vi "Timer1 Callback.vi"   [LabVIEW 2014]
doc: "Callback VI for the timer interrupt."
uses:
  <vilib>/Aledyne-TSXperts/Arduino Compatible Compiler for LabVIEW/Arduino Compatible Compiler for LabVIEW.lvlib
  Timer1/Timer1.lvlib
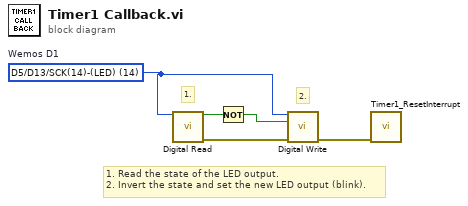
[diagram p0: block diagram]
diagram:
  w1 = u8 14 items=["D0-RX(3)"=3, "D1-TX(1)"=1, "D2(16)"=16, "D3/D15/SCL(5)"=5, "D4/D14/SDA(4)"=4, "D5/D13/SCK(14)-(LED)"=14, "D6/D12/MISO(12)"=12, "D7/D11/MOSI(13)"=13, "D8(0)"=0, "D9/TX1(2)"=2, "D10/SS (15)"=15, "ADC0,(17)"=17]  # Wemos D1
  # "2."
  # "1."
  # "1. Read the state of the LED output.\n2. Invert the state and set the new LED output (blink)."
  n1 = call <vilib>:"Digital Read.vi"("pin"=w1) -> ("state"=w5:bool, "error out"=w3:errorcluster)  [unwired: 13 in]
  n2 = Not(x=w5) -> (.not. x?=w4:bool)
  n3 = call <vilib>:"Digital Write.vi"("pin"=w1, "state"=w4, "error in (no error)"=w3) -> ("error out"=w2:errorcluster)  [unwired: 12 in]
  n4 = call "Timer1_ResetInterrupt.vi"("error in"=w2) -> ()  [unwired: 10 in, 1 out]
